vi "from string.vi"(8 "error in":errorcluster, 9 "data":string, 10 "version":string, 11 "FPGA Module configuration in":refnum<class "FPGA Module configuration.lvclass">) -> (0 "error out":errorcluster, 3 "FPGA Module configuration out":refnum<class "FPGA Module configuration.lvclass">)   [LabVIEW 2014, in "FPGA Module configuration.lvclass"]
doc: "Provides an interface for loading a module configuration from a file or other serialized data source. It is recommended that all children of this class store data in two sets--data required for its own initialization, and any data required for parent initialization--and that each implementation uses the <b>Call Parent Method</b> primitive to de-serialize parent information. As a result, it is expected that every module configuration class calls <b>component configuration.lvclass:From String.vi</b>."
uses:
  FPGA Module configuration.lvclass
  Line.ctl
  fpga channel/FPGA Channel.lvclass
  FPGA Module configuration.lvclass/FPGA Module configuration.ctl
  <vilib>/NI/Tag Bus Module Framework/module configuration/TBM module configuration.lvclass
  <vilib>/NI/Configuration Framework/serializable configuration/NISE_CEF_serializable configuration.lvclass
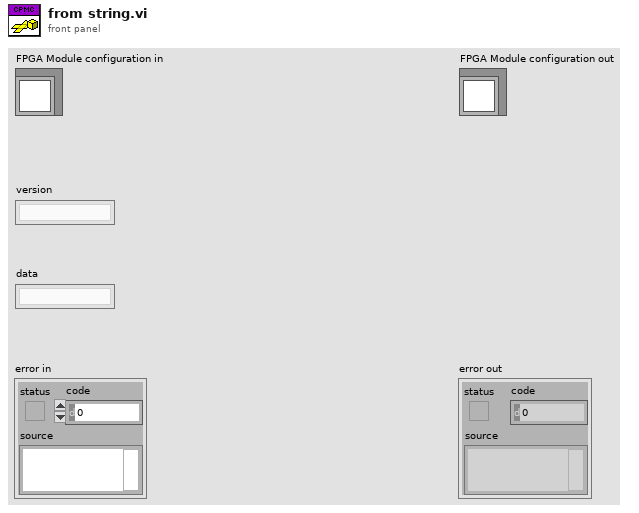
[diagram p1: front panel]
types:
  T1 = typedef "FPGA Module configuration.lvclass/Line.ctl" = cluster{"Channel":refnum<class "FPGA Channel.lvclass">}
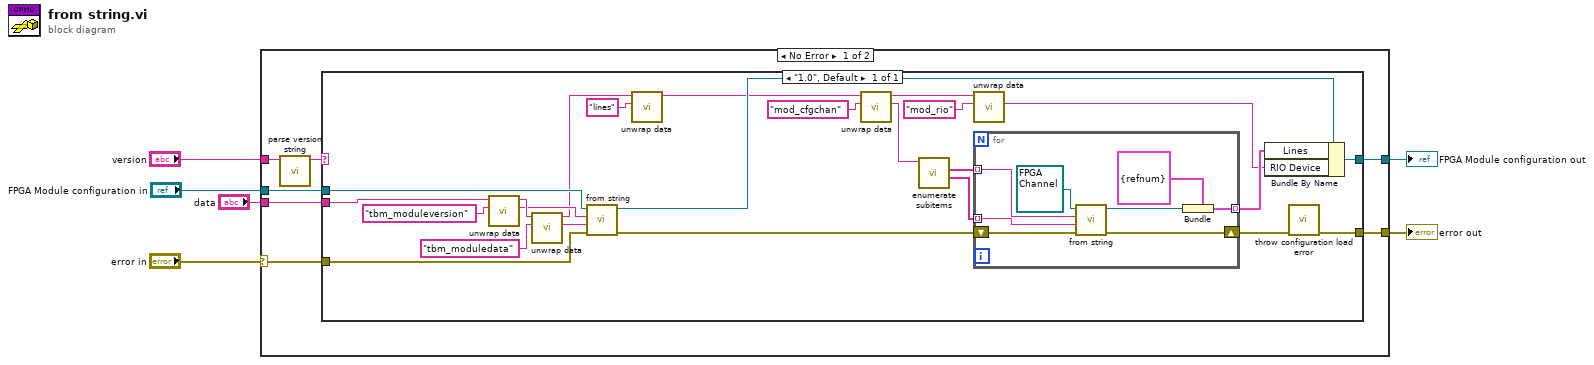
[diagram p0: block diagram]
diagram:
  n1 = case shown="No Error" "error in" {
    selector: "error in" -> [w7 w47]
    tunnel: "data" -> [w13 _]
    tunnel: "FPGA Module configuration in" -> [w12 w46]
    tunnel: [w11 w46] -> w5
    tunnel: [w10 w47] -> w4
    tunnel: "version" -> [w9 _]
    frame No Error {
      n2 = call <vilib>:"parse version string.vi"("full version"=w9) -> ("major.minor version"=w8:string)  [unwired: 7 in, 3 out]
      n3 = case shown="\"1.0\", Default" w8 {
        tunnel: w13 -> [w34]
        tunnel: w7 -> [w33]
        tunnel: w12 -> [w37]
        tunnel: [w25] -> w11
        tunnel: [w36] -> w10
        frame "1.0", Default {
          n4 = call <vilib>:"unwrap data.vi"("identifier"="tbm_moduleversion" ("additional identifier"), "data to unwrap"=w34) -> ("unwrapped data"=w29:string, "remaining string"=w35:string)  [unwired: 8 in]
          n5 = call <vilib>:"unwrap data.vi"("identifier"="tbm_moduledata" ("additional identifier"), "data to unwrap"=w35) -> ("unwrapped data"=w31:string, "remaining string"=w28:string)  [unwired: 8 in]
          n6 = call-parent "from string.vi"("error in"=w33, "data"=w31, "version"=w29, "module configuration in"=w37) -> ("error out"=w20:errorcluster, "module configuration out"=w26:refnum<class "FPGA Module configuration.lvclass">)  [unwired: 6 in]
          n7 = call <vilib>:"unwrap data.vi"("identifier"="lines" ("additional identifier"), "data to unwrap"=w28) -> ("remaining string"=w24:string)  [unwired: 8 in, 1 out]
          n8 = call <vilib>:"unwrap data.vi"("identifier"="mod_cfgchan", "data to unwrap"=w24) -> ("unwrapped data"=w19:string, "remaining string"=w16:string)  [unwired: 8 in]
          n9 = call <vilib>:"enumerate subitems.vi"("data to enumerate"=w19) -> ("associated data"=w21:string[], "discovered subitems"=w22:string[])  [unwired: 8 in, 1 out]
          n10 = call <vilib>:"unwrap data.vi"("identifier"="mod_rio", "data to unwrap"=w16) -> ("unwrapped data"=w14:string)  [unwired: 8 in, 1 out]
          n11 = for {
            shift-right: [w45] -> w17
            shift-left: w20 -> [w44]
            tunnel: w22 -> [w43] mode=indexing
            tunnel: w21 -> [w42] mode=indexing
            tunnel: [w39] -> w18 mode=indexing
            n12 = call-dynamic "from string.vi"("error in"=w44, "channel data"=w42, "identifier"=w43, "channel in"=refnum<class "FPGA Channel.lvclass"> refnum ("FPGA Channel.lvclass")) -> ("error out"=w45:errorcluster, "channel out"=w40:refnum<class "FPGA Channel.lvclass">)  [unwired: 6 in]
            n13 = Bundle(cluster=T1 {"Channel"=refnum} ("Line"), "Channel"=w40) -> (w39:T1)
          }
          n14 = Bundle By Name(cluster=w26, "Lines"=w18, "RIO Device"=w14) -> (w25:refnum<class "FPGA Module configuration.lvclass">)
          n15 = call <vilib>:"throw configuration load error.vi"("error in"=w17) -> ("error out"=w36:errorcluster)  [unwired: 10 in]
        }
      }
    }
    frame Error {
    }
  }
  "error out" <- w4
  "FPGA Module configuration out" <- w5
